vi "WPI_AnalogChannelSetAveraging.vi"(8 "error in (no error)":errorcluster, 9 "OversampleBits":u8=10, 10 "AverageBits":u8, 11 "AIDeviceRef":T1={"DevStatus"={"status"=FALSE, "code"=0, "source"=""}, "Analog Channel"=enum."Invalid"}) -> (0 "error out":errorcluster, 3 "AIDeviceRef":T1={"DevStatus"={"status"=FALSE, "code"=0, "source"=""}, "Analog Channel"=enum."Invalid"})   [LabVIEW 2017]
doc: "Specifies the number of bits you want to use to average and oversample the signal. Averaging can improve measurement accuracy for noisy and rapidly changing signals. Oversampling is a technique that sums extra samples but does not divide the sum by the number of samples. For example, if you oversample a signal by 16 times, the resulting values are 16 times larger than the average output. Use oversampling to improve the resolution of signal measurements at the expense of the sampling rate. The FPGA on the CompactRIO device automatically does the oversampling.\n\nThis software is licensed. Open the labview\\readme\\WPI Robotics Library Open Source License.txt file for more information."
uses:
  <vilib>/Rock Robotics/WPI/AnalogChannel/WPI_AnalogChannelDevRef.ctl
  <vilib>/Rock Robotics/SystemInterfaces/AI/FPGA_AIChannel.ctl
  <vilib>/Rock Robotics/SystemInterfaces/System/FPGA_SystemGet.vi
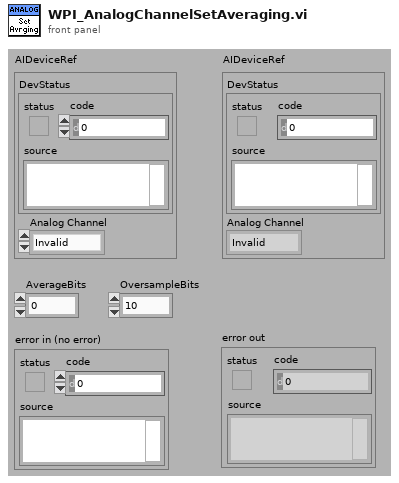
[diagram p1: front panel]
types:
  T1 = typedef "WPI_AnalogChannelDevRef.ctl" = cluster{"DevStatus":errorcluster, "Analog Channel":T2}
  T2 = typedef "FPGA_AIChannel.ctl" = enum8{"AI 0", "AI 1", "AI 2", "AI 3", "AI MXP 0", "AI MXP 1", "AI MXP 2", "AI MXP 3", "Invalid"}
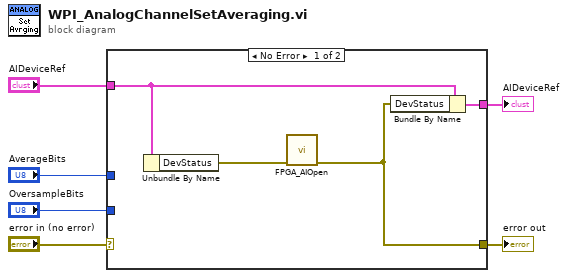
[diagram p0: block diagram]
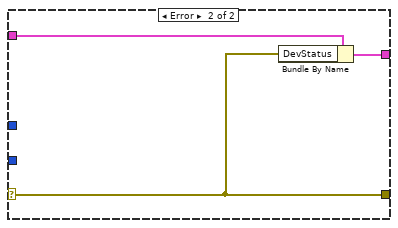
[diagram p2: hidden frame]
diagram:
  n1 = case shown="No Error" "error in (no error)" {
    selector: "error in (no error)" -> [_ w11]
    tunnel: [w9 w13] -> w6
    tunnel: "AIDeviceRef" -> [w8 w12]
    tunnel: [w7 w11] -> w3
    tunnel: "AverageBits" -> [_ _]
    tunnel: "OversampleBits" -> [_ _]
    frame No Error {
      n2 = Unbundle By Name(w8) -> ("DevStatus"=w10:errorcluster)
      n3 = call <vilib>:"FPGA_AIOpen.vi"("error in (no error)"=w10) -> ("error out"=w7:errorcluster)  [unwired: 2 in, 8 out]
      n4 = Bundle By Name(cluster=w8, "DevStatus"=w7) -> (w9:T1)
    }
    frame Error {
      n5 = Bundle By Name(cluster=w12, "DevStatus"=w11) -> (w13:T1)
    }
  }
  "AIDeviceRef" <- w6
  "error out" <- w3
